vi "ITX2 Plot Commands.vi"(1 "X,Y Log":i32[](array[numeric]), 4 "Plot labels":string[](array[string])=["time", "V", "V^2", "V^3"], 5 "X,Y Labels":string[](array[string])=["x label", "y label"], 6 "wavenames":string[](array[string])=["time.datatest.000005", "V.datatest.000005", "V^2.datatest.000005", "V^3.datatest.000005"]) -> (0 "result string":string="Display/R 'time.datatest.000005'\nAppendToGraph 'V.datatest.000005'\nAppendToGraph 'V^2.datatest.000005'\nAppendToGraph 'V^3.datatest.000005'\nLabel bottom \"x label\"\nLabel left \"y label\"\nModifyGraph rgb('time.datatest.000005')=(65280,0,0)\nModifyGraph rgb('V.datatest.000005')=(41984,65280,0)\nModifyGraph rgb('V^2.datatest.000005')=(0,65280,45568)\nModifyGraph rgb('V^3.datatest.000005')=(2048,0,65280)\nLegend/C/N=text0/J \"\\\\s('time.datatest.000005') time\\r\\\\s('V.datatest.000005') V\\r\\\\s('V^2.datatest.000005') V^2\\r\\\\s('V^3.datatest.000005') V^3\"\nModifyGraph mirror=1\nModifyGraph width=216\nModifyGraph height={Aspect,0.6}\nModifyGraph Log(bottom)=0\nModifyGraph Log(left)=0\n")   [LabVIEW 2016, in "LV-Data.ITX.lvclass"]
uses:
  LV-Data.ITX.lvclass
  ITX Commands/typedefs/Label--cluster.ctl
  ITX Commands/typedefs/Log--cluster.ctl
  ITX Commands/typedefs/log--enum.ctl
  ITX Commands/ITX Commands.lvclass
panel:
  # "Legend/C/N=text0/J \"\\\\s('y_test.000011Plot9') Plot 9\\r\\\\s('y_test.000011Plot8') Plot 8\""
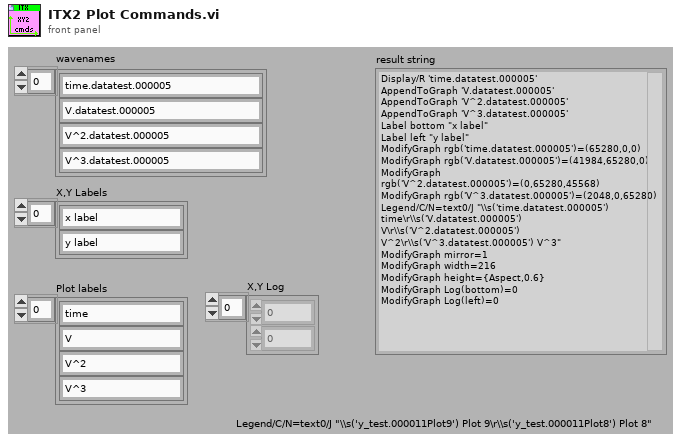
[diagram p1: front panel]
types:
  T1 = typedef "ITX Commands.lvclass/Log--cluster.ctl" = cluster{"bottom":T2, "left":T2}
  T2 = typedef "ITX Commands.lvclass/log--enum.ctl" = enum16{"normal axis", "log base 10", "log base 2"}
  T3 = typedef "ITX Commands.lvclass/Label--cluster.ctl" = cluster{"Bottom":string, "Top":string, "Left":string, "Right":string}
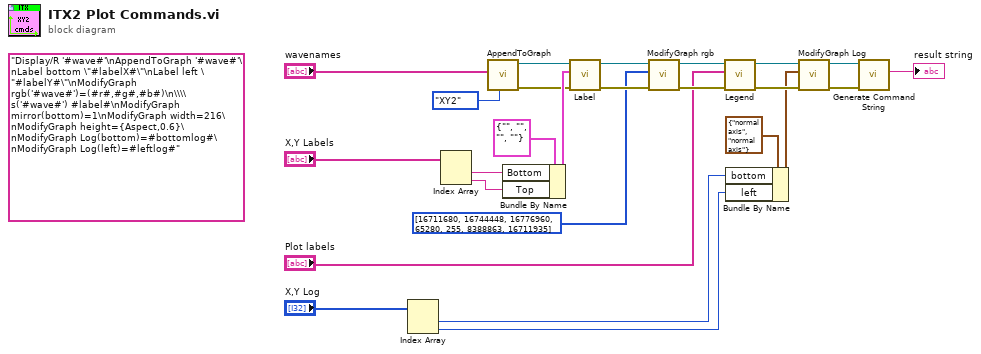
[diagram p0: block diagram]
diagram:
  (unwired) "Display/R '#wave#'\nAppendToGraph '#wave#'\nLabel bottom \"#labelX#\"\nLabel left \"#labelY#\"\nModifyGraph rgb('#wave#')=(#r#,#g#,#b#)\n\\\\s('#wave#') #label#\nModifyGraph mirror(bottom)=1\nModifyGraph width=216\nModifyGraph height={Aspect,0.6}\nModifyGraph Log(bottom)=#bottomlog#\nModifyGraph Log(left)=#leftlog#" ("input string")
  n1 = Index Array(array="X,Y Log") -> (element #1=w3:i32, element #2=w5:i32)  [unwired: 2 in]
  n2 = Index Array(array="X,Y Labels") -> (element #1=w20:string, element #2=w2:string)  [unwired: 2 in]
  n3 = call "AppendToGraph.vi"("Enum"=enum16{"XY", "XY2"}."XY2", "wavenames"="wavenames") -> ("error out"=w19:errorcluster, "ITX Commands out"=w21:refnum<class "ITX Commands.lvclass">)  [unwired: 8 in]
  n4 = Bundle By Name(cluster=T3 {"Bottom"="", "Top"="", "Left"="", "Right"=""} ("Label"), "Bottom"=w20, "Top"=w2) -> (w22:T3)
  n5 = call "Label.vi"("error in (no error)"=w19, "Label"=w22, "ITX Commands in"=w21) -> ("error out"=w17:errorcluster, "ITX Commands out"=w18:refnum<class "ITX Commands.lvclass">)  [unwired: 7 in]
  n6 = call "ModifyGraph rgb.vi"("error in (no error)"=w17, "Colorscale"=u32[] [16711680, 16744448, 16776960, 65280, 255, 8388863, 16711935], "ITX Commands in"=w18) -> ("error out"=w15:errorcluster, "ITX Commands out"=w14:refnum<class "ITX Commands.lvclass">)  [unwired: 7 in]
  n7 = call "Legend.vi"("error in (no error)"=w15, "Plot labels"="Plot labels", "ITX Commands in"=w14) -> ("error out"=w11:errorcluster, "ITX Commands out"=w10:refnum<class "ITX Commands.lvclass">)  [unwired: 7 in]
  n8 = Bundle By Name(cluster=T1 {"bottom"=enum."normal axis", "left"=enum."normal axis"} ("Log"), "bottom"=w3, "left"=w5) -> (w6:T1)
  n9 = call "ModifyGraph Log.vi"("error in (no error)"=w11, "Log"=w6, "ITX Commands in"=w10) -> ("error out"=w8:errorcluster, "ITX Commands out"=w9:refnum<class "ITX Commands.lvclass">)  [unwired: 7 in]
  n10 = call "Generate Command String.vi"("ITX Commands in"=w9, "error in (no error)"=w8) -> ("ITX Commands"=→"result string":string)  [unwired: 6 in, 2 out]
